vi "Read ID.vi"(8 "error in (no error)":errorcluster, 11 "client in":refnum<class "client.lvclass">) -> (0 "error out":errorcluster, 2 "ID":string, 3 "client out":refnum<class "client.lvclass">)   [LabVIEW 2016, in "client.lvlib" / "client.lvclass"]
uses:
  client.lvclass
  client.lvclass/client.ctl
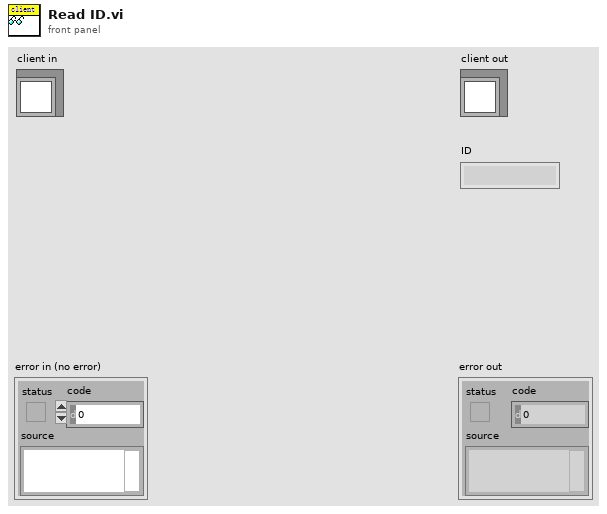
[diagram p1: front panel]
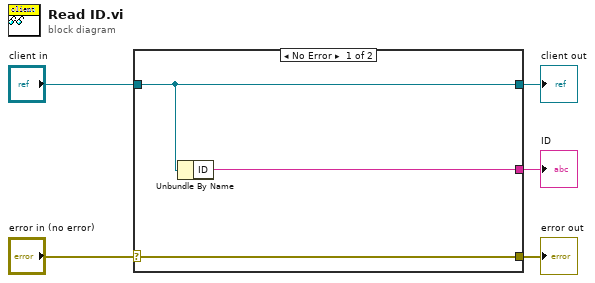
[diagram p0: block diagram]
diagram:
  n1 = case shown="No Error" "error in (no error)" {
    selector: "error in (no error)" -> [w8 w9]
    tunnel: [w8 w9] -> w4
    tunnel: [w7 w10] -> w2
    tunnel: "client in" -> [w7 w10]
    tunnel: [w6 _] -> w1
    frame No Error {
      n2 = Unbundle By Name(w7) -> ("ID"=w6:string)
    }
    frame Error {
    }
  }
  "error out" <- w4
  "client out" <- w2
  "ID" <- w1
